vi "hokuyo_largestHole.vi"(1 "Current stepper angle":dbl, 2 "Array":cluster{"Magnitude":dbl, "Direction":dbl}[](array[cluster])) -> (0 "Target Direction":dbl)   [LabVIEW 2014]
panel:
  out "Hole Size":dbl
  in  "stop":bool
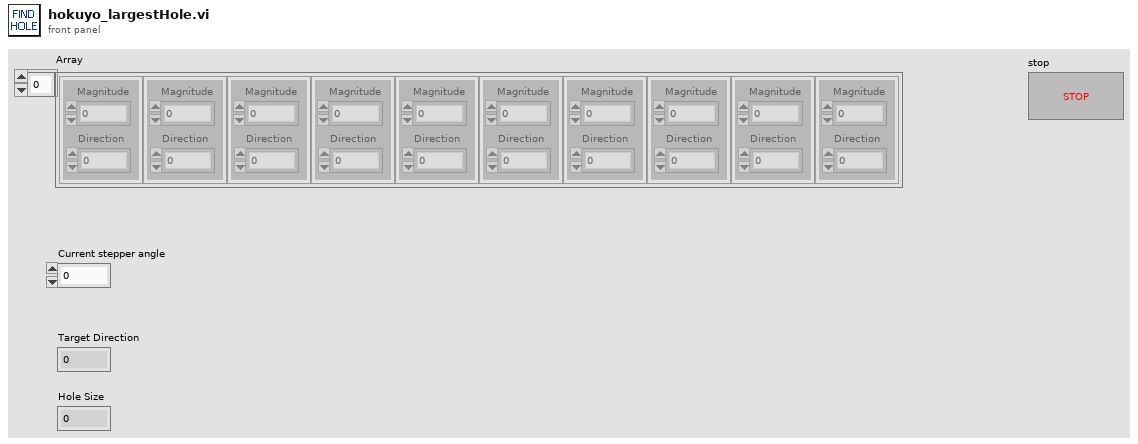
[diagram p1: front panel]
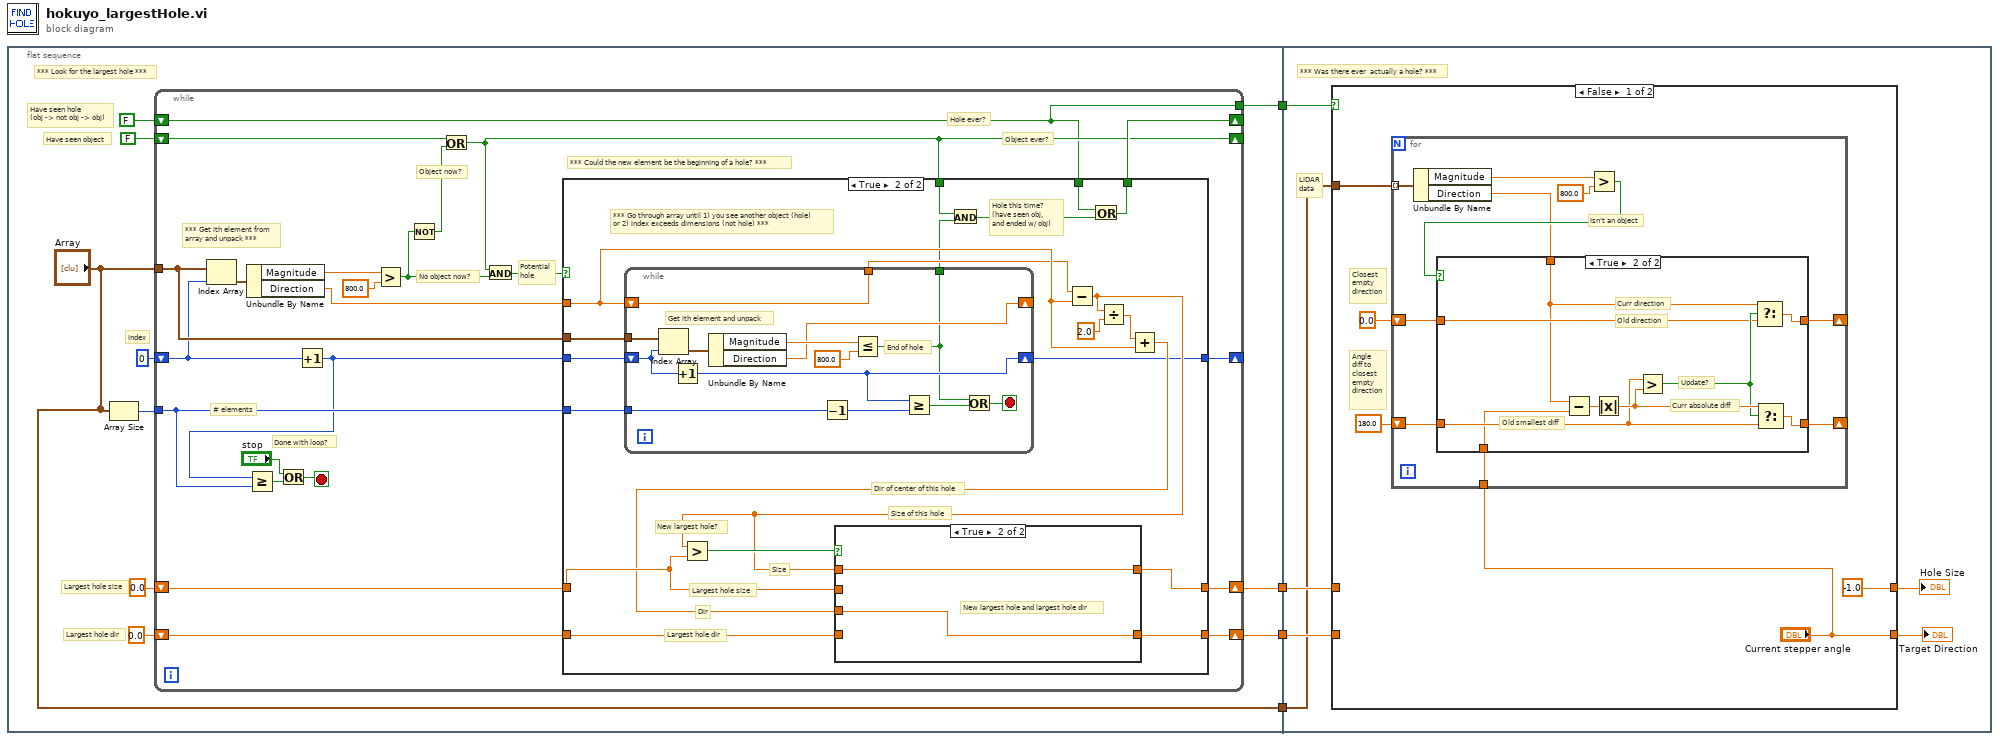
[diagram p0: block diagram]
diagram:
  n1 = flat-sequence {
    tunnel: [w8] -> w4
    tunnel: [w7] -> w3
    tunnel: ["Array"] -> w2
    tunnel: [w5] -> w1
    tunnel: w4 -> [w84]
    tunnel: w3 -> [w83]
    tunnel: w2 -> [w80]
    tunnel: w1 -> [w79]
    frame #0 {
      # "*** Look for the largest hole ***"
      # "Index"
      # "Have seen hole\n(obj -> not obj -> obj)"
      # "Have seen object"
      # "Largest hole dir"
      # "Largest hole size"
      n2 = Array Size(array="Array") -> (size(s)=w11:i32)
      n3 = while {
        tunnel: "Array" -> [w35]
        shift-right: [w36] -> _
        shift-left: 0 -> [w28]
        shift-right: [w20] -> w8
        shift-left: 0.0 -> [w33]
        shift-right: [w19] -> w7
        shift-left: 0.0 ("Largest Hole Direction") -> [w34]
        tunnel: w11 -> [w27]
        shift-right: [w17] -> _
        shift-left: FALSE -> [w24]
        shift-right: [w21] -> _
        shift-left: FALSE -> [w15]
        tunnel: [w15] -> w5
        stop <- w32 stop-if-true
        # "# elements"
        # "Hole ever?"
        # "Object ever?"
        # "Potential\nhole"
        # "Object now?"
        # "No object now?"
        # "Done with loop?"
        # "*** Could the new element be the beginning of a hole? ***"
        # "*** Get ith element from \narray and unpack ***"
        n4 = Index Array(array=w35, index=w28) -> (element=w37:cluster{"Magnitude":dbl, "Direction":dbl})
        n5 = Unbundle By Name(w37) -> ("Magnitude"=w25:dbl, "Direction"=w18:dbl)
        n6 = Increment(x=w28) -> (x+1=w16:i32)
        n7 = Greater Or Equal?(x=w16, y=w27) -> (x >= y?=w31:bool)
        n8 = Or(x="stop", y=w31) -> (x .or. y?=w32:bool)
        n9 = Greater?(x=w25, y=800.0) -> (0:w23:bool)
        n10 = Not(x=w23) -> (.not. x?=w22:bool)
        n11 = Or(x=w24, y=w22) -> (x .or. y?=w17:bool)
        n12 = And(x=w17, y=w23) -> (x .and. y?=w26:bool)
        n13 = case shown="True" w26 {
          tunnel: w16 -> [w41 w61]
          tunnel: [w41 w50] -> w36
          tunnel: w35 -> [_ w60]
          tunnel: w18 -> [_ w48]
          tunnel: w34 -> [w40 w54]
          tunnel: w33 -> [w39 w58]
          tunnel: [w40 w52] -> w19
          tunnel: [w39 w53] -> w20
          tunnel: w27 -> [_ w49]
          tunnel: w15 -> [w38 w46]
          tunnel: [w38 w45] -> w21
          tunnel: w17 -> [_ w42]
          frame False {
            # "*** Keep looking for the beginning of a hole ***"
          }
          frame True {
            # "Hole this time? \n(have seen obj,\nand ended w/ obj)"
            # "Largest hole size"
            # "Size"
            # "Largest hole dir"
            # "Dir"
            # "New largest hole?"
            # "Dir of center of this hole"
            # "Size of this hole"
            # "*** Go through array until 1) you see another object (hole) \nor 2) index exceeds dimensions (not hole) ***"
            n14 = while {
              tunnel: w60 -> [w78]
              shift-right: [w72] -> w50
              shift-left: w61 -> [w74]
              tunnel: w49 -> [w66]
              shift-right: [w70] -> _
              shift-left: w48 -> [w69]
              tunnel: [w69] -> w47
              tunnel: [w68] -> w43
              stop <- w73 stop-if-true
              # "Get ith element and unpack"
              # "End of hole"
              n15 = Index Array(array=w78, index=w74) -> (element=w75:cluster{"Magnitude":dbl, "Direction":dbl})
              n16 = Increment(x=w74) -> (x+1=w72:i32)
              n17 = Unbundle By Name(w75) -> ("Magnitude"=w76:dbl, "Direction"=w70:dbl)
              n18 = Decrement(x=w66) -> (x-1=w67:i32)
              n19 = Less Or Equal?(x=w76, y=800.0) -> (x <= y?=w68:bool)
              n20 = Greater Or Equal?(x=w72, y=w67) -> (x >= y?=w71:bool)
              n21 = Or(x=w68, y=w71) -> (x .or. y?=w73:bool)
            }
            n22 = And(x=w42, y=w43) -> (x .and. y?=w44:bool)
            n23 = Subtract(x=w47, y=w48) -> (x-y=w51:dbl)
            n24 = Greater?(x=w51, y=w58) -> (0:w59:bool)
            n25 = Or(x=w46, y=w44) -> (x .or. y?=w45:bool)
            n26 = Divide(x=w51, y=2.0) -> (x/y=w56:dbl)
            n27 = Add(x=w56, y=w48) -> (x+y=w55:dbl)
            n28 = case shown="True" w59 {
              tunnel: w58 -> [w63 _]
              tunnel: w55 -> [_ w65]
              tunnel: w54 -> [w62 _]
              tunnel: [w63 w64] -> w53
              tunnel: [w62 w65] -> w52
              tunnel: w51 -> [_ w64]
              frame False {
                # "Keep old largest hole and largest hole dir"
              }
              frame True {
                # "New largest hole and largest hole dir"
              }
            }
          }
        }
      }
    }
    frame #1 {
      # "LIDAR\ndata"
      # "*** Was there ever  actually a hole? ***"
      n29 = case shown="False" w79 {
        tunnel: w84 -> [_ w112]
        tunnel: w83 -> [_ w111]
        tunnel: [-1.0 w112] -> w82
        tunnel: ["Current stepper angle" w111] -> w81
        tunnel: w80 -> [w89 _]
        frame False {
          # "Angle\ndiff to\nclosest\nempty\ndirection"
          # "Closest\nempty \ndirection"
          n30 = for {
            tunnel: w89 -> [w99] mode=indexing
            shift-right: [w91] -> _
            shift-left: 0.0 -> [w94]
            shift-right: [w92] -> _
            shift-left: 180.0 -> [w93]
            tunnel: "Current stepper angle" -> [w90]
            # "Isn't an object"
            n31 = Unbundle By Name(w99) -> ("Magnitude"=w98:dbl, "Direction"=w95:dbl)
            n32 = Greater?(x=w98, y=800.0) -> (0:w96:bool)
            n33 = case shown="True" w96 {
              tunnel: w95 -> [_ w105]
              tunnel: w94 -> [w100 w106]
              tunnel: w93 -> [w101 w103]
              tunnel: [w101 w107] -> w92
              tunnel: [w100 w104] -> w91
              tunnel: w90 -> [_ w102]
              frame False {
                # "Don't update if it's an object, not empty space"
              }
              frame True {
                # "Curr direction"
                # "Old direction"
                # "Curr absolute diff"
                # "Old smallest diff"
                # "Update?"
                n34 = Subtract(x=w105, y=w102) -> (x-y=w110:dbl)
                n35 = Absolute Value(x=w110) -> (abs(x)=w109:dbl)
                n36 = Greater?(x=w103, y=w109) -> (0:w108:bool)
                n37 = Select(t=w105, s=w108, f=w106) -> (s? t:f=w104:dbl)
                n38 = Select(t=w109, s=w108, f=w103) -> (s? t:f=w107:dbl)
              }
            }
          }
        }
        frame True {
          # "Yes, there was a hole - use values from previous panel"
        }
      }
      "Target Direction" <- w81
      "Hole Size" <- w82
    }
  }
